vi "UpdateAlbum.vi"(8 "error in":errorcluster, 9 "Album Index":i32, 10 "AlbumArray":T1, 11 "UI Refs":T2) -> (0 "error out":errorcluster, 1 "Album Index":string)   [LabVIEW 2015]
uses:
  Controls & Type Defs/UI Data.ctl
  Controls & Type Defs/AlbumArray.ctl
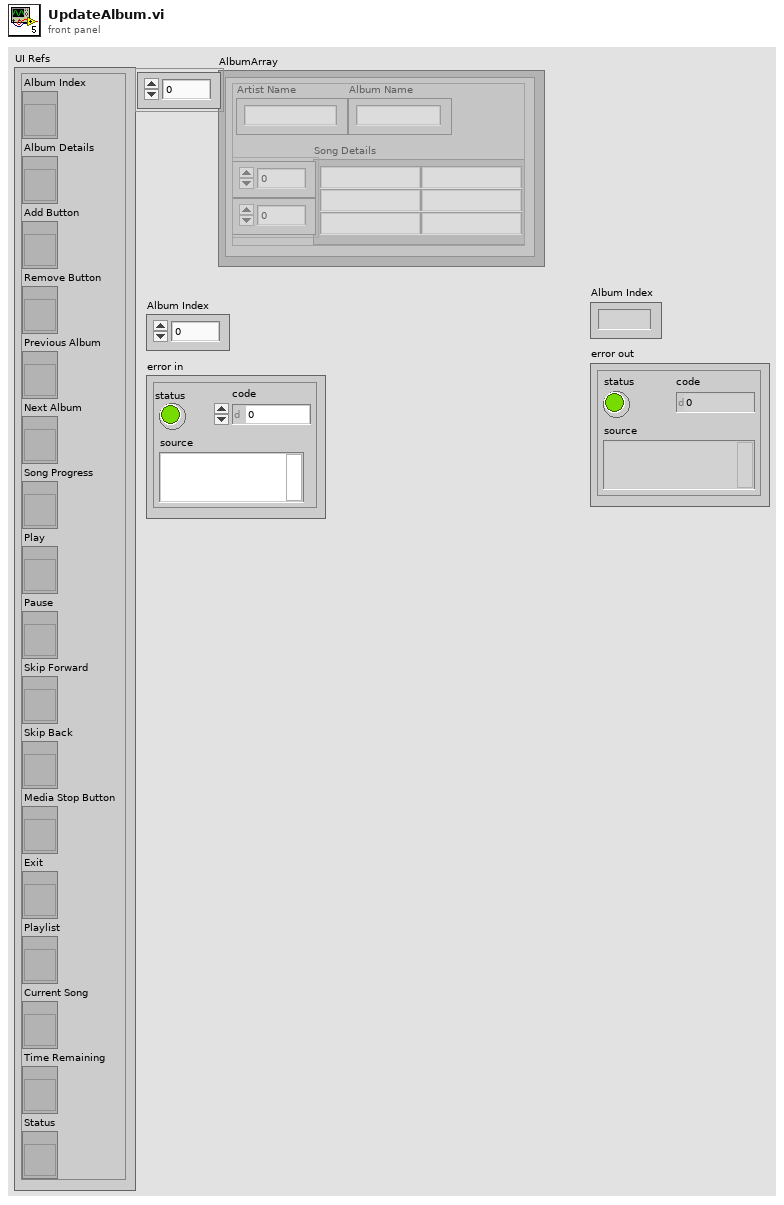
[diagram p1: front panel]
types:
  T1 = typedef "AlbumArray.ctl" = cluster{"Artist Name":string, "Album Name":string, "Song Details":string[][]}[]
  T2 = typedef "UI Data.ctl" = cluster{"Album Index":refnum<vi>, "Album Details":refnum<vi>, "Add Button":refnum<vi>, "Remove Button":refnum<vi>, "Previous Album":refnum<vi>, "Next Album":refnum<vi>, "Song Progress":refnum<vi>, "Play":refnum<vi>, "Pause ":refnum<vi>, "Skip Forward":refnum<vi>, "Skip Back":refnum<vi>, "Media Stop Button":refnum<vi>, "Exit":refnum<vi>, "Playlist":refnum<vi>, "Current Song":refnum<vi>, "Time Remaining":refnum<vi>, "Status":refnum<vi>}
  T3 = cluster{"Artist Name":string, "Album Name":string, "Song Details":string[][]}
  T4 = typedef "AlbumDetails.ctl" = cluster{"Artist":string, "Album Name":string, "Songs":i32}
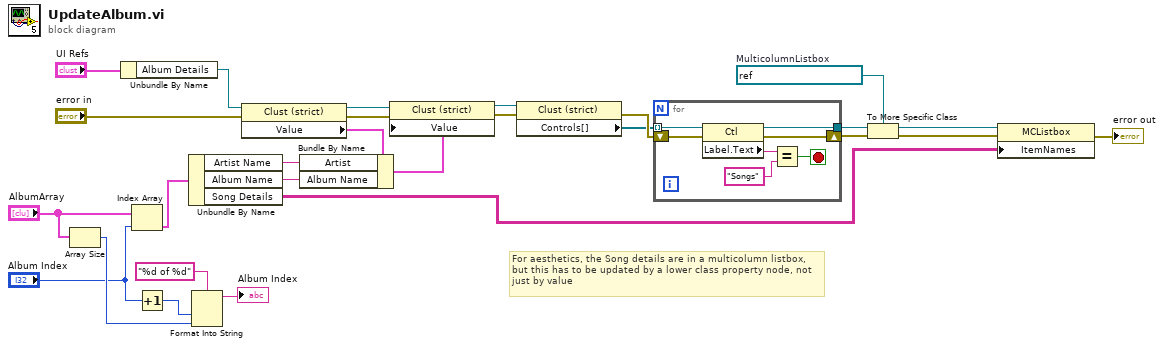
[diagram p0: block diagram]
diagram:
  w24 = refnum<vi> refnum  # MulticolumnListbox
  # "For aesthetics, the Song details are in a multicolumn listbox, but this has to be updated by a lower class property node, not just by value"
  n1 = Array Size(array="AlbumArray") -> (size(s)=w4:i32)
  n2 = Unbundle By Name("UI Refs") -> ("Album Details"=w16:refnum<vi>)
  n3 = Index Array(array="AlbumArray", index="Album Index") -> (element=w5:T3)
  n4 = Increment(x="Album Index") -> (x+1=w6:i32)
  n5 = Unbundle By Name(w5) -> ("Artist Name"=w14:string, "Album Name"=w15:string, "Song Details"=w1:string[][])
  n6 = Format Into String(format string="%d of %d", w6, w4) -> (resulting string=→"Album Index":string)  [unwired: 2 in, 1 out]
  n7 = property class="Clust (strict)"(reference=w16, error in="error in") -> (reference out=w10:refnum<vi>, error out=w11:errorcluster, "Value"=w13:T4)
  n8 = Bundle By Name(cluster=w13, "Artist"=w14, "Album Name"=w15) -> (w27:T4)
  n9 = property class="Clust (strict)"(reference=w10, error in=w11, "Value"=w27) -> (reference out=w17:refnum<vi>, error out=w23:errorcluster)
  n10 = property class="Clust (strict)"(reference=w17, error in=w23) -> (error out=w22:errorcluster, "Controls[]"=w18:refnum<vi>[])  [unwired: 1 out]
  n11 = for {
    tunnel: w18 -> [w34] mode=indexing
    tunnel: [w33] -> w19
    shift-right: [w29] -> w21
    shift-left: w22 -> [w28]
    stop <- w30 stop-if-true
    n12 = property class="Ctl"(reference=w34, error in=w28) -> (reference out=w33:refnum<vi>, error out=w29:errorcluster, "Label.Text"=w31:string)
    n13 = Equal?(x=w31, y="Songs") -> (x = y?=w30:bool)
  }
  n14 = To More Specific Class(target class=w24, reference=w19, error in=w21) -> (specific class reference=w20:refnum<vi>, error out=w25:errorcluster)
  n15 = property class="MCListbox"(reference=w20, error in=w25, "ItemNames"=w1) -> (error out=→"error out":errorcluster)  [unwired: 1 out]
